vi "AtSpectrograph_monitorCommand_start.vi"(8 "error in (no error)":errorcluster, 11 "command_start_Ctl":T1) -> (0 "error out":errorcluster, 2 "function return":i32, 3 "command_start_Ctl out":T1)   [LabVIEW 2016, in "SALLV_AtSpectrograph.lvlib"]
doc: "int AtSpectrograph_shm_monitorCommand_startLV(AtSpectrograph_command_startLV *command_start_Ctl );"
uses:
  SALLV_AtSpectrograph.lvlib
  DataTypes/command_start.ctl
  SALLV_AtSpectrograph.so
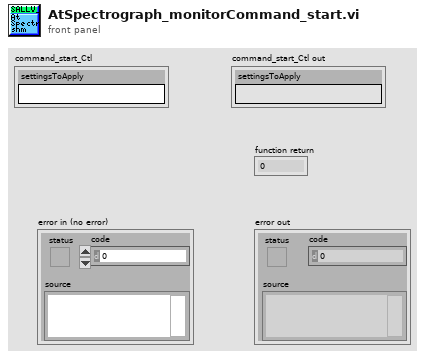
[diagram p1: front panel]
types:
  T1 = typedef "SALLV_AtSpectrograph.lvlib/command_start.ctl" = cluster{"settingsToApply":string}
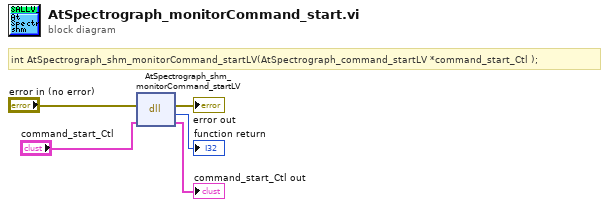
[diagram p0: block diagram]
diagram:
  # "int AtSpectrograph_shm_monitorCommand_startLV(AtSpectrograph_command_startLV *command_start_Ctl );"
  n1 = dll-call lib="home/harini/tcs/temp/SALLV_AtSpectrograph/SALLV_AtSpectrograph.*" fn="AtSpectrograph_shm_monitorCommand_startLV"(error in="error in (no error)", "command_start_Ctl"="command_start_Ctl") -> (error out=→"error out":errorcluster, →"function return":i32, "command_start_Ctl"=→"command_start_Ctl out":T1)  [unwired: 2 in, 1 out]
